vi "Error Handl_Write Error Info File.vi"(8 "error in":errorcluster caption="错误输入", 10 "Error Info":string, 11 "Error log file":path) -> (0 "error out":errorcluster caption="错误输出")   [LabVIEW 2016]
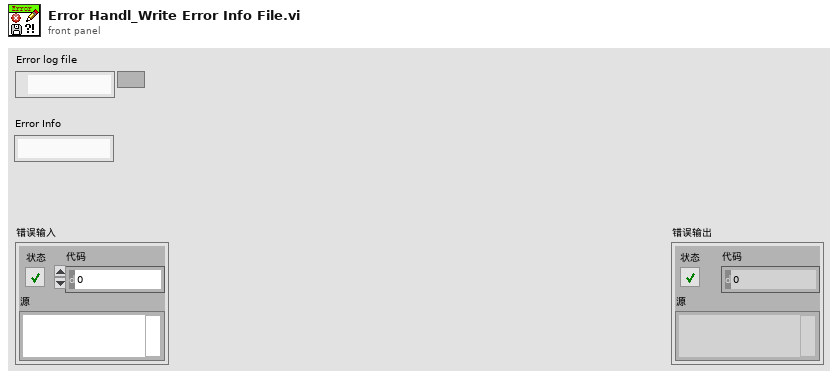
[diagram p1: front panel]
types:
  T1 = enum16{"open", "replace", "create", "open or create", "replace or create", "replace or create with confirmation"}
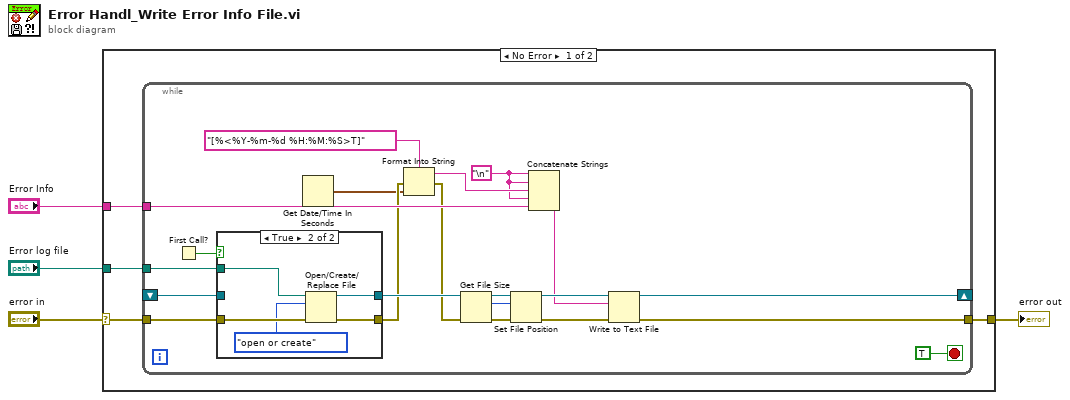
[diagram p0: block diagram]
diagram:
  n1 = case shown="No Error" "error in" {
    selector: "error in" -> [w8 w37]
    tunnel: [w5 w37] -> w3
    tunnel: "Error log file" -> [w7 _]
    tunnel: "Error Info" -> [w6 _]
    frame No Error {
      n2 = while {
        tunnel: w8 -> [w26]
        tunnel: w7 -> [w27]
        shift-right: [w24] -> _
        shift-left: _ -> [w25]
        tunnel: w6 -> [w17]
        tunnel: [w10] -> w5
        stop <- TRUE stop-if-true
        w9 = "\n"
        n3 = First Call?() -> (First Call?: T/F=w28:bool)
        n4 = case shown="True" w28 {
          tunnel: w27 -> [_ w36]
          tunnel: w26 -> [w30 w35]
          tunnel: [w31 w33] -> w23
          tunnel: w25 -> [w31 _]
          tunnel: [w30 w32] -> w16
          frame False {
          }
          frame True {
            n5 = Open/Create/Replace File(file path (use dialog)=w36, error in=w35, operation (0:open)=T1."open or create" ("操作(0:open)")) -> (refnum out=w33:refnum<file>, error out=w32:errorcluster)  [unwired: 3 in, 1 out]
          }
        }
        n6 = Get Date/Time In Seconds() -> (seconds since 1Jan1904=w13:timestamp)
        n7 = Format Into String(format string="[%<%Y-%m-%d %H:%M:%S>T]" ("格式字符串"), error in=w16, w13) -> (resulting string=w12:string, error out=w15:errorcluster)  [unwired: 1 in]
        n8 = Get File Size(file=w23, error in=w15) -> (refnum out=w22:refnum<file>, size (in bytes)=w19:i64, 0:w20:errorcluster)
        n9 = Set File Position(offset (in bytes) (0)=w19, refnum=w22, error in=w20) -> (refnum out=w21:refnum<file>, error out=w18:errorcluster)  [unwired: 1 in]
        n10 = Concatenate Strings(w9, w9, w12, w9, w17) -> (w11:string)
        n11 = Write to Text File(file (use dialog)=w21, text=w11, error in=w18) -> (refnum out=w24:refnum<file>, error out=w10:errorcluster)  [unwired: 1 in, 1 out]
      }
    }
    frame Error {
    }
  }
  "error out" <- w3
